vi "GetCXT.vi"(5 "format string (%_20f)":string="%_20f", 7 "key description":string, 8 "sections":string[](array[string]), 9 "numeric":cxt, 11 "info data":string) -> (0 "sections out":string[](array[string]), 1 "found?":bool, 2 "value":cxt format="%#_20g", 3 "info data out":string)   [LabVIEW 2013, in "infolib.lvlib"]
doc: "Add a new numeric key to Info Data string. If section exists in Info Data string, inserts key into this section."
uses:
  infolib.lvlib
panel:
  out "value 3":ext
  out "value 2":ext
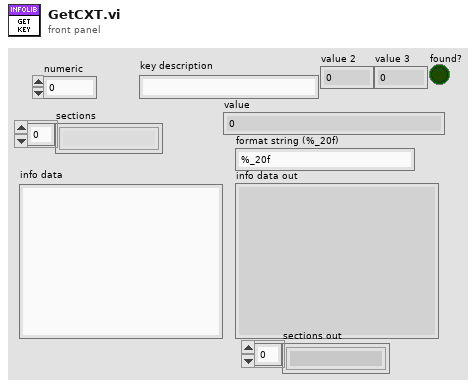
[diagram p1: front panel]
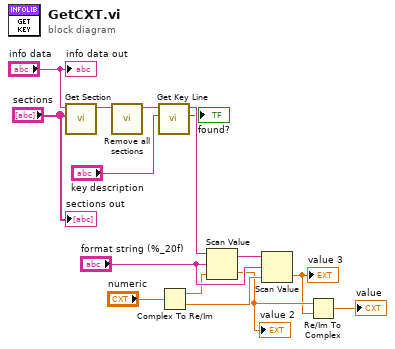
[diagram p0: block diagram]
diagram:
  n1 = call "Get Section.vi"("sections"="sections", "info data"="info data") -> ("section part"=w15:string)  [unwired: 8 in, 1 out]
  n2 = call "Remove all sections.vi"("info data"=w15) -> ("info data out"=w13:string)  [unwired: 10 in]
  n3 = call "Get Key Line.vi"("key description"="key description", "info data"=w13) -> ("found?"=→"found?":bool, "key value"=w10:string)  [unwired: 8 in]
  n4 = Complex To Re/Im(x + iy="numeric") -> (x=w6:ext, y=w5:ext)
  n5 = Scan Value(string=w10, format string="format string (%_20f)", default (0 dbl)=w6) -> (output string=w9:string, value=w4:ext)
  "value 2" <- w4
  n6 = Scan Value(string=w9, format string="format string (%_20f)", default (0 dbl)=w5) -> (value=w3:ext)  [unwired: 1 out]
  "value 3" <- w3
  n7 = Re/Im To Complex(1:w3, 2:w4) -> (0:→"value":cxt)
  "info data out" <- "info data"
  "sections out" <- "sections"
